vi "DuplicateTaskItem.vi"(10 "TaskConfig":refnum<data-value>, 11 "Task":string) -> ()   [LabVIEW 2025, in "DAQ_Module.lvlib" / "DAQ_Module.lvclass"]
uses:
  DAQ_Module.lvclass
  DAQ_Config.ctl
  DAQ_Task_Config.ctl
  DAQ_HW_Type.ctl
  DAQ_Task_Type.ctl
  DAQ_SampleRateConfig.ctl
  DAQ_Module.lvclass/DAQ_Module.ctl
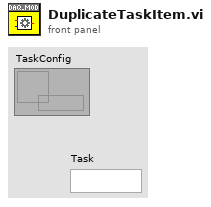
[diagram p1: front panel]
types:
  T1 = typedef "DAQ_Module.lvlib/DAQ_Module.lvclass/DAQ_Config.ctl" = map{string, T2}
  T2 = typedef "DAQ_Module.lvlib/DAQ_Module.lvclass/DAQ_Task_Config.ctl" = cluster{"Drive":T3, "TaskType":T4, "PhysicalChannels":string, "SampleRateConfiguration":T5, "ChannelConfig":map{string, cluster{"Name":string, "Config":string}}, "Enable":bool, "ShowPanel":bool}
  T3 = typedef "DAQ_Module.lvlib/DAQ_Module.lvclass/DAQ_HW_Type.ctl" = enum16{"NI_DAQmx", "Simulated_DAQ"}
  T4 = typedef "DAQ_Module.lvlib/DAQ_Module.lvclass/DAQ_Task_Type.ctl" = enum16{"AI", "Linear", "Angular", "AO"}
  T5 = typedef "DAQ_Module.lvlib/DAQ_Module.lvclass/DAQ_SampleRateConfig.ctl" = cluster{"SampleRate":dbl, "SamplesPerChannel":u32, "SamplesPerRead":i32, "SampleMode":i32, "Clock Source":string}
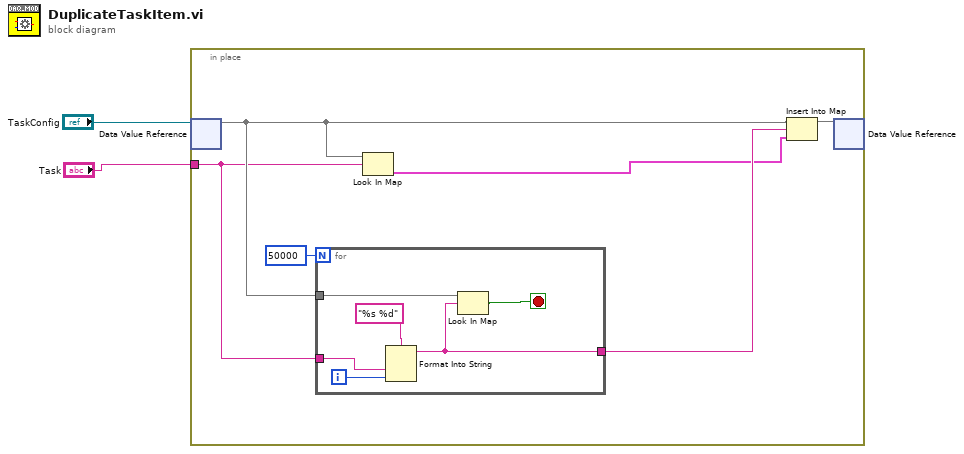
[diagram p0: block diagram]
diagram:
  n1 = in-place {
    in-place-border: "Task" -> [w4]
    n2 = in-place-dvr #1("TaskConfig") -> (w5:T1)  [unwired: 1 out]
    n3 = for {
      N: 50000 -> [_]
      tunnel: w5 -> [w14]
      tunnel: [w11] -> w7
      tunnel: w4 -> [w10]
      i -> [w9]
      stop <- w13 stop-if-true
      n4 = Format Into String(format string="%s %d", w10, w9) -> (resulting string=w11:string)  [unwired: 2 in, 1 out]
      n5 = Look In Map(map=w14, key=w11) -> (key not found?=w13:bool)  [unwired: 1 in, 1 out]
    }
    n6 = Look In Map(map=w5, key=w4) -> (value=w3:T2)  [unwired: 1 in, 1 out]
    n7 = Insert Into Map(map in=w5, key=w7, value=w3) -> (map out=w6:T1)  [unwired: 2 out]
    n8 = in-place-dvr #1(w6) -> ()  [unwired: 2 out]
  }
